vi "Intensity-color-maping.vi"() -> ()   [LabVIEW 2020]
uses:
  <vilib>/imath/engines/lvmath2/RunTimeEngine/Managers/WorkSpace/UID Generator.vi
  <vilib>/imath/engines/lvmath2/RunTimeEngine/BuiltInFunctions/timerstart/NIMS_timerstart.vi
  <vilib>/imath/engines/lvmath2/RunTimeEngine/BuiltInFunctions/linramp/NIMS_linramp.vi
  <vilib>/imath/engines/lvmath2/RunTimeEngine/BuiltInFunctions/meshgrid2d/NIMS_meshgrid2d(V,V).vi
  <instcachedir>/0/NIMS_meshgrid2d(V,V)_3733343E1C554A708015CFB0432C6A59.lvgen/NIMS_meshgrid2d(V,V)_3733343E1C554A708015CFB0432C6A59_000.vi
  <vilib>/imath/engines/lvmath2/RunTimeEngine/ArithmeticOperatorToken/NIMS_ArithmeticOperator_plus.vi
  <instcachedir>/0/NIMS_ArithmeticOperator_plus_54468E2FAC2848C4BF0D457641184E60.lvgen/NIMS_ArithmeticOperator_plus_54468E2FAC2848C4BF0D457641184E60_010.vi
  <vilib>/imathl/engines/lvmath/Functions/Error Handling/Create Error.vi
  <vilib>/imath/engines/lvmath2/RunTimeEngine/RangeToken/NIMS_Range_R2 - Integer.vi
  <instcachedir>/0/NIMS_Range_R2 - Integer_FFC1A4B1B9F04947ABCB56F009996D55.lvgen/NIMS_Range_R2 - Integer_FFC1A4B1B9F04947ABCB56F009996D55_000.vi
  <vilib>/imath/engines/lvmath2/RunTimeEngine/CommandStatement/MC_CommandStatement_break.vi
  <vilib>/imath/engines/lvmath2/RunTimeEngine/ArithmeticOperatorToken/NIMS_ArithmeticOperator_power(S).vi
  <instcachedir>/0/NIMS_ArithmeticOperator_power(S)_0FB4C2FA3CD746849DC4699515FAC284.lvgen/NIMS_ArithmeticOperator_power(S)_0FB4C2FA3CD746849DC4699515FAC284_012.vi
  <instcachedir>/0/NIMS_ArithmeticOperator_plus_54468E2FAC2848C4BF0D457641184E60.lvgen/NIMS_ArithmeticOperator_plus_54468E2FAC2848C4BF0D457641184E60_002.vi
  <vilib>/imath/engines/lvmath2/RunTimeEngine/ErrorHandling/NIMS_Create Error From Enums.vi
  <vilib>/imath/engines/lvmath2/RunTimeEngine/BuiltInFunctions/abs/NIMS_abs(signed).vi
  <instcachedir>/0/NIMS_abs(signed)_C4FCB8E6058B49B797C7C8D53CA5F6EC.lvgen/NIMS_abs(signed)_C4FCB8E6058B49B797C7C8D53CA5F6EC_003.vi
  <vilib>/imath/engines/lvmath2/RunTimeEngine/BuiltInFunctions/timerstop/NIMS_timerstop.vi
  <vilib>/imath/engines/lvmath2/RunTimeEngine/Managers/SymbolTable/Clear UID.vi
  <vilib>/imath/engines/lvmath2/RunTimeEngine/NodeEndStatement/NIMS_NodeEndStatement_Output.vi
  <instcachedir>/0/NIMS_NodeEndStatement_Output_53EC0D466D134D7ABD903AC30B43404B.lvgen/NIMS_NodeEndStatement_Output_53EC0D466D134D7ABD903AC30B43404B_001.vi
  <instcachedir>/0/NIMS_NodeEndStatement_Output_53EC0D466D134D7ABD903AC30B43404B.lvgen/NIMS_NodeEndStatement_Output_53EC0D466D134D7ABD903AC30B43404B_002.vi
  <vilib>/imath/engines/lvmath2/RunTimeEngine/ErrorHandling/NIMS_Finalize Error.vi
  <vilib>/imath/engines/lvmath2/RunTimeEngine/Managers/SymbolTable/NIMS_WorkSpace.lvlib
panel:
  out "Fractal Plot":dbl[][](graph)
  out "Calculation Time (sec)":dbl caption="Calculation Time [sec]"
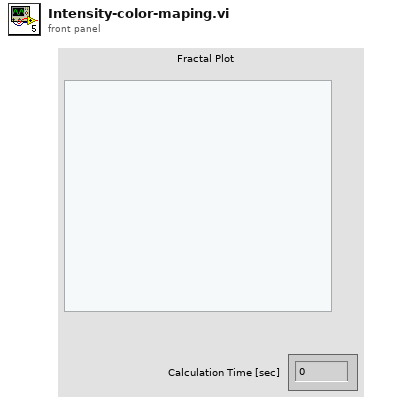
[diagram p1: front panel]
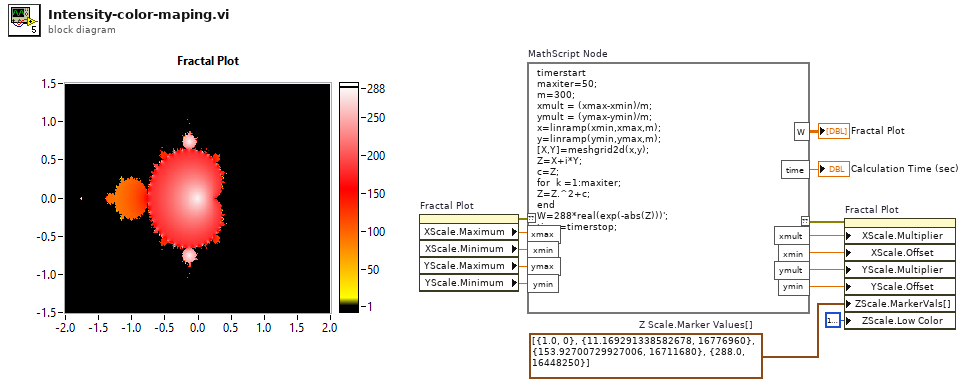
[diagram p0: block diagram]
diagram:
  w6 = cluster{dbl, u32}[] [{1.0, 0}, {11.169291338582678, 16776960}, {153.92700729927006, 16711680}, {288.0, 16448250}]  # Z Scale.Marker Values[]
  n1 = property on="Fractal Plot" class="IntGraph (strict)"() -> (error out=w8:errorcluster, "XScale.Maximum"=w12:dbl, "XScale.Minimum"=w11:dbl, "YScale.Maximum"=w10:dbl, "YScale.Minimum"=w9:dbl)  [unwired: 2 in, 1 out]
  n2 = mathscript code="timerstart\nmaxiter=50;\nm=300;\nxmult = (xmax-xmin)/m;\nymult = (ymax-ymin)/m;\nx=linramp(xmin,xmax,m);\ny=linramp(ymin,ymax,m);\n[X,Y]=meshgrid2d(x,y);\nZ=X+i*Y;\nc=Z;\nfor  k =1:maxiter;\nZ=Z.^2+c;\nend\nW=288*real(exp(-abs(Z)))';\ntime=timerstop;"("??"=w8, "xmax"=w12, "xmin"=w11, "ymax"=w10, "ymin"=w9) -> ("??"=w1:errorcluster, "W"=→"Fractal Plot":dbl[][], "time"=→"Calculation Time (sec)":dbl, "xmin"=w3:dbl, "xmult"=w2:dbl, "ymin"=w5:dbl, "ymult"=w4:dbl)
  n3 = property on="Fractal Plot" class="IntGraph (strict)"(error in=w1, "XScale.Multiplier"=w2, "XScale.Offset"=w3, "YScale.Multiplier"=w4, "YScale.Offset"=w5, "ZScale.MarkerVals[]"=w6, "ZScale.Low Color"=u32 16777222 ("Plot Area:Colors:BG Color")) -> ()  [unwired: 1 in, 2 out]
